vi "数组操作.vi"(9 "操作码":dbl, 10 "输入点":cluster{"x":dbl, "y":dbl}, 11 "数组输入":cluster{"x":dbl, "y":dbl}[](array[cluster])) -> (1 "索引":dbl, 2 "输出点":cluster{"x":dbl, "y":dbl}, 3 "数组输出":cluster{"x":dbl, "y":dbl}[](array[cluster]))   [LabVIEW 2012]
panel:
  # "0：插入末尾\n1：删除开头\n2：查找输入"
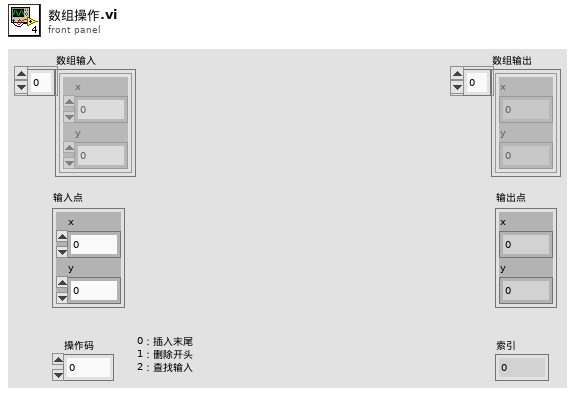
[diagram p1: front panel]
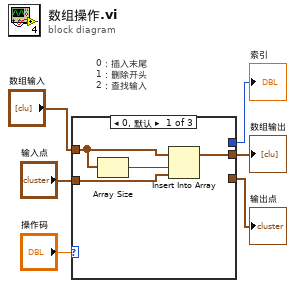
[diagram p0: block diagram]
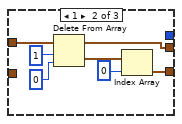
[diagram p2: hidden frame]
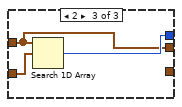
[diagram p3: hidden frame]
diagram:
  # "0：插入末尾\n1：删除开头\n2：查找输入"
  n1 = case shown="0, 默认" "操作码" {
    tunnel: "数组输入" -> [w10 w17 w18]
    tunnel: "输入点" -> [w9 _ w20]
    tunnel: [w7 w14 w18] -> w3
    tunnel: [_ w11 _] -> w2
    tunnel: [_ _ w19] -> w1
    frame 0, Default {
      n2 = Array Size(array=w10) -> (size(s)=w8:i32)
      n3 = Insert Into Array(array=w10, index=w8, new element=w9) -> (w7:cluster{"x":dbl, "y":dbl}[])
    }
    frame 1 {
      n4 = Delete From Array(array=w17, length=1 ("长度"), index=0 ("索引")) -> (deleted portion=w13:cluster{"x":dbl, "y":dbl}[], array with subset deleted=w14:cluster{"x":dbl, "y":dbl}[])
      n5 = Index Array(array=w13, index=0 ("索引")) -> (element=w11:cluster{"x":dbl, "y":dbl})
    }
    frame 2 {
      n6 = Search 1D Array(1D array=w18, element=w20) -> (index of element=w19:i32)  [unwired: 1 in]
    }
  }
  "数组输出" <- w3
  "索引" <- w1
  "输出点" <- w2
